vi "Convert Channel Values to PWM Generate Digital Settings.vi"(9 "Length":i32, 10 "Index":i32, 11 "Channel Values in":dbl[](array[numeric])) -> (2 "PWM Generate Digital Settings":T1, 3 "Channel Values out":dbl[](array[numeric]))   [LabVIEW 2018, in "FPGA Addon Engine.lvlib"]
uses:
  FPGA Addon Engine.lvlib
  Submodules/Source/Types/PWM.Generate.Digital.Settings.ctl
  Submodules/Source/Speciality FPGA IO.lvlib
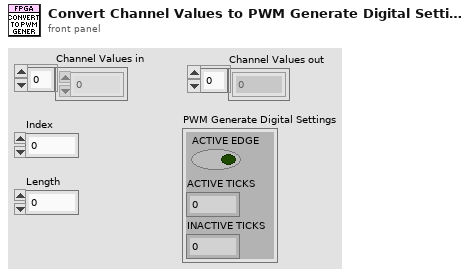
[diagram p1: front panel]
types:
  T1 = typedef "Speciality FPGA IO.lvlib/PWM.Generate.Digital.Settings.ctl" = cluster{"ACTIVE EDGE":bool, "ACTIVE TICKS":u32, "INACTIVE TICKS":u32}
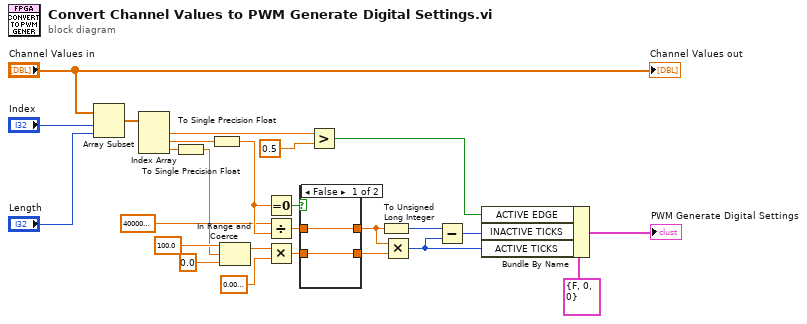
[diagram p0: block diagram]
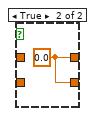
[diagram p2: hidden frame]
diagram:
  n1 = Array Subset(array="Channel Values in", index="Index", length="Length") -> (w4:dbl[])
  n2 = Index Array(array=w4) -> (element #1=w7:dbl, element #2=w9:dbl, element #3=w8:dbl)  [unwired: 3 in]
  n3 = To Single Precision Float(number=w8) -> (single precision float=w16:sgl)
  n4 = To Single Precision Float(number=w9) -> (single precision float=w15:sgl)
  n5 = In Range and Coerce(upper limit=sgl 100.0, x=w16, lower limit=sgl 0.0) -> (coerced(x)=w17:sgl)  [unwired: 1 out]
  n6 = Equal To 0?(x=w15) -> (x = 0?=w10:bool)
  n7 = Divide(x=sgl 40000000.0 ("y"), y=w15) -> (x/y=w12:sgl)
  n8 = Multiply(x=w17, y=sgl 0.01 ("x")) -> (x*y=w14:sgl)
  n9 = case shown="False" w10 {
    tunnel: [w28 w29] -> w11
    tunnel: w12 -> [w28 _]
    tunnel: [w27 w29] -> w13
    tunnel: w14 -> [w27 _]
    frame False {
    }
    frame True {
      w29 = sgl 0.0
    }
  }
  n10 = Greater?(x=w7, y=0.5) -> (0:w6:bool)
  n11 = To Unsigned Long Integer(number=w11) -> (unsigned 32bit integer=w2:u32)
  n12 = Multiply(x=w11, y=w13) -> (x*y=w23:u32)
  n13 = Subtract(x=w2, y=w23) -> (x-y=w22:u32)
  n14 = Bundle By Name(cluster=T1 {"ACTIVE EDGE"=FALSE, "ACTIVE TICKS"=0, "INACTIVE TICKS"=0} ("Settings"), "ACTIVE EDGE"=w6, "INACTIVE TICKS"=w22, "ACTIVE TICKS"=w23) -> (→"PWM Generate Digital Settings":T1)
  "Channel Values out" <- "Channel Values in"
